vi "Dynamic Get TestSuite Test Paths.vi"(8 "error in":errorcluster, 11 "Test Project":path) -> (0 "error out":errorcluster, 3 "Test Paths":path[](array[path]))   [LabVIEW 2011, in "GraphicalTestRunner.lvlib"]
uses:
  GraphicalTestRunner.lvlib
  Get TestSuite Test Paths.vi
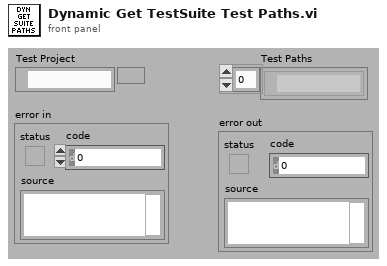
[diagram p1: front panel]
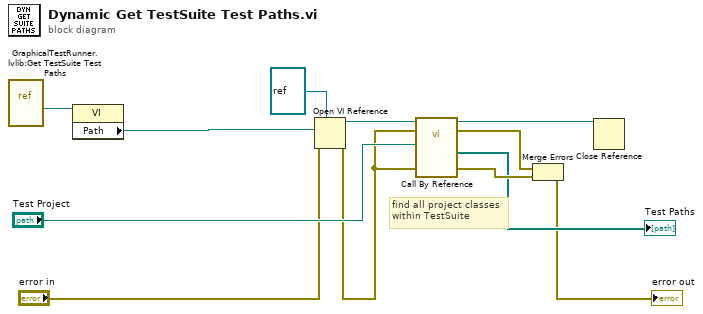
[diagram p0: block diagram]
diagram:
  # "find all project classes\nwithin TestSuite"
  n1 = vi-ref "GraphicalTestRunner.lvlib:Get TestSuite Test Paths.vi"() -> (w1:refnum<vi>)
  n2 = property class="VI"(reference=w1) -> ("Path"=w5:path)  [unwired: 1 in, 2 out]
  n3 = Open VI Reference(type specifier VI Refnum (for type only)=refnum<vi> refnum, vi path=w5, error in (no error)="error in") -> (vi reference=w11:refnum<vi>, error out=w3:errorcluster)  [unwired: 3 in]
  n4 = call-by-ref "?"(reference=w11, error in=w3, 8:"error in (no error)"=w3, "Test Project"="Test Project") -> (reference out=w2:refnum<vi>, error out=w10:errorcluster, 0:"error out"=w9:errorcluster, "Test Paths"=→"Test Paths":path[])  [unwired: 8 in]
  n5 = Merge Errors(w10, w9) -> (→"error out":errorcluster)
  n6 = Close Reference(reference=w2) -> ()  [unwired: 1 in, 1 out]
